vi "VI Tree - appcontrol__ogtk.vi"() -> ()   [LabVIEW 2012]
uses:
  <userlib>/_OpenG.lib/appcontrol/appcontrol.llb/ClassID Names Enum__ogtk.ctl
panel:
  in  "paths":T1
  in  "VI Refnum":refnum<vi>
  in  "Gen Refnum Array 2":refnum<vi>[](array[refnum])
  in  "Gen Refnum Array":refnum<vi>[](array[refnum])
  in  "Gen Refnum":refnum<vi>
  out "ClassID Name":T2=enum."Decoration"
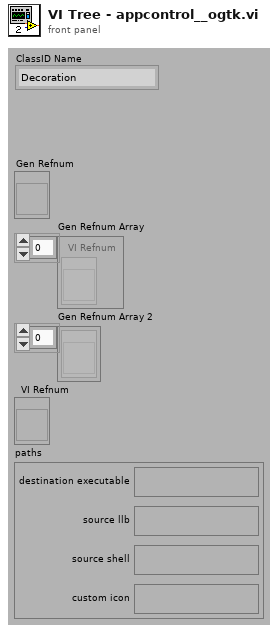
[diagram p1: front panel]
types:
  T1 = cluster{"destination executable":path, "source llb":path, "source shell":path, "custom icon":path}
  T2 = typedef "ClassID Names Enum__ogtk.ctl" = enum32{"0 <undefined>", "1 <undefined>", "2 <undefined>", "Generic", "Decoration", "Text", "Control", "ColorBox", "Boolean", "RefNum", "Variant", "Path", "ListBox", "Table", "Array", "Picture", "ActiveXContainer", "Numeric", "Digital", "NamedNumeric", "ColorRamp", "Slide", "GraphOrChart", "WaveformChart", "WaveformGraph", "IntensityChart", "IntensityGraph", "String", "IOName", "ComboBox", "Cluster", "Panel", "Knob", "NumWithScale", "Ring", "Enum", "GObject", "Plot", "Cursor", "NumericText", "Scale", "ColorScale", "GraphScale", "ColorGraphScale", "TypedRefNum", "OldKnobScale", "MCListbox", "MeasureData", "BVTag", "DAQName", "VISAName", "IVIName", "SlideScale", "TabControl", "Page", "TabArrayTabControl", "ConPane"}
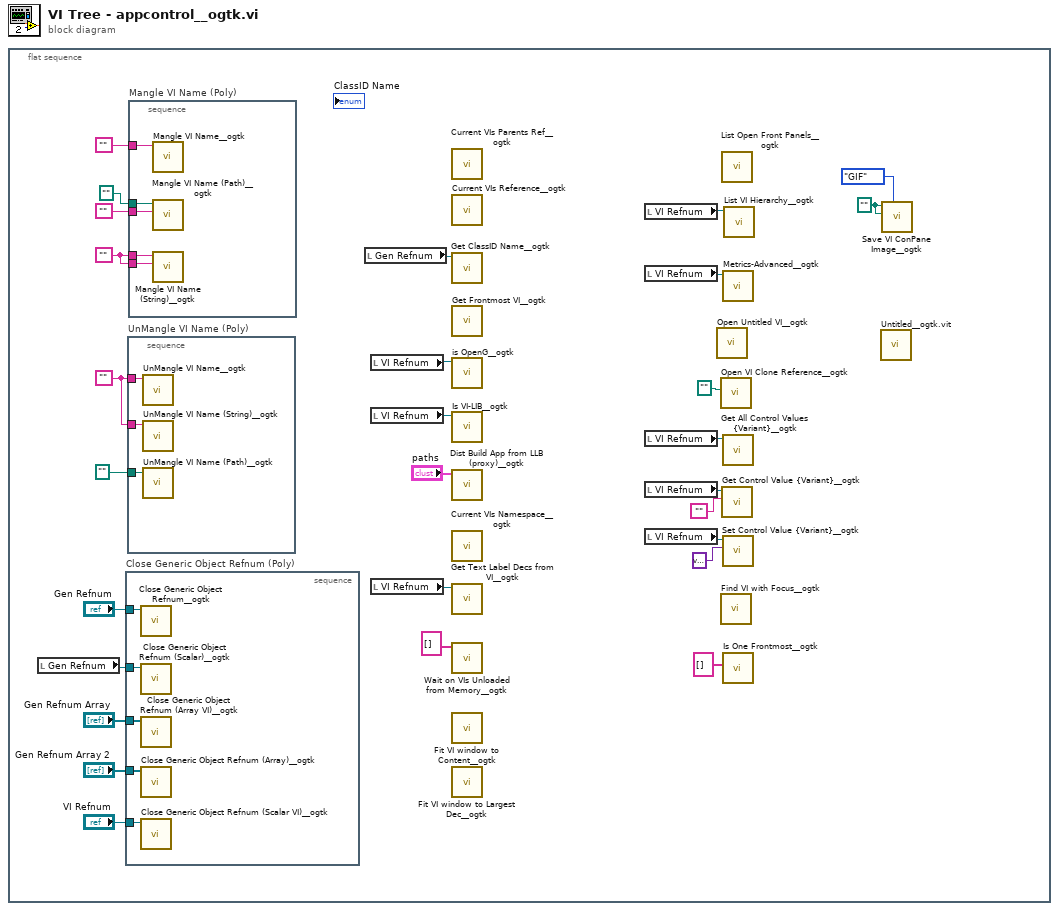
[diagram p0: block diagram]
diagram:
  n1 = flat-sequence {
    frame #0 {
      w2 = path ""
      w18 = ""
      w27 = ""
      n2 = local read "Gen Refnum"() -> (w14:refnum<vi>)
      n3 = stacked-sequence "Close Generic Object Refnum (Poly)" {
        tunnel: "Gen Refnum" -> [w36]
        tunnel: "Gen Refnum Array" -> [w35]
        tunnel: "Gen Refnum Array 2" -> [w34]
        tunnel: "VI Refnum" -> [w33]
        tunnel: w14 -> [w32]
        frame #0 {
          n4 = call-poly <userlib>:"Close Generic Object Refnum__ogtk.vi"("Gen Refnum"=w36) -> ()  [unwired: 10 in, 1 out]
          n5 = call <userlib>:"Close Generic Object Refnum (Scalar)__ogtk.vi"("Gen Refnum"=w32) -> ()  [unwired: 10 in, 1 out]
          n6 = call <userlib>:"Close Generic Object Refnum (Array VI)__ogtk.vi"("Gen Refnum Array"=w35) -> ()  [unwired: 9 in, 2 out]
          n7 = call <userlib>:"Close Generic Object Refnum (Array)__ogtk.vi"("Gen Refnum Array"=w34) -> ()  [unwired: 10 in, 1 out]
          n8 = call <userlib>:"Close Generic Object Refnum (Scalar VI)__ogtk.vi"("VI Refnum"=w33) -> ()  [unwired: 9 in, 2 out]
        }
      }
      n9 = stacked-sequence "UnMangle VI Name (Poly)" {
        tunnel: w27 -> [w31]
        tunnel: path "" -> [w30]
        tunnel: w27 -> [w29]
        frame #0 {
          n10 = call-poly <userlib>:"UnMangle VI Name__ogtk.vi"("Mangled Name"=w29) -> ()  [unwired: 8 in, 3 out]
          n11 = call <userlib>:"UnMangle VI Name (String)__ogtk.vi"("Mangled Name"=w31) -> ()  [unwired: 8 in, 3 out]
          n12 = call <userlib>:"UnMangle VI Name (Path)__ogtk.vi"("Mangled Name"=w30) -> ()  [unwired: 8 in, 3 out]
        }
      }
      n13 = stacked-sequence "Mangle VI Name (Poly)" {
        tunnel: "" -> [w41]
        tunnel: "" -> [w40]
        tunnel: path "" -> [w39]
        tunnel: w18 -> [w38]
        tunnel: w18 -> [w37]
        frame #0 {
          n14 = call-poly <userlib>:"Mangle VI Name__ogtk.vi"("Name"=w41) -> ()  [unwired: 9 in, 2 out]
          n15 = call <userlib>:"Mangle VI Name (Path)__ogtk.vi"("Namespace (\"\": don't mangle)"=w40, "Name"=w39) -> ()  [unwired: 8 in, 2 out]
          n16 = call <userlib>:"Mangle VI Name (String)__ogtk.vi"("Namespace (\"\": don't mangle)"=w37, "Name"=w38) -> ()  [unwired: 8 in, 2 out]
        }
      }
      n17 = local read "Gen Refnum"() -> (w15:refnum<vi>)
      n18 = local read "VI Refnum"() -> (w13:refnum<vi>)
      n19 = local read "VI Refnum"() -> (w12:refnum<vi>)
      n20 = local read "VI Refnum"() -> (w17:refnum<vi>)
      n21 = call <userlib>:"Current VIs Parents Ref__ogtk.vi"() -> ()  [unwired: 2 in, 1 out]
      n22 = call <userlib>:"Current VIs Reference__ogtk.vi"() -> ()  [unwired: 5 in, 1 out]
      n23 = call <userlib>:"Get ClassID Name__ogtk.vi"("Gen Refnum"=w15) -> ()  [unwired: 7 in, 4 out]
      n24 = call <userlib>:"Get Frontmost VI__ogtk.vi"() -> ()  [unwired: 1 out]
      n25 = call <userlib>:"is OpenG__ogtk.vi"("VI reference"=w13) -> ()  [unwired: 8 in, 3 out]
      n26 = call <userlib>:"Is VI-LIB__ogtk.vi"("VI reference"=w12) -> ()  [unwired: 8 in, 3 out]
      n27 = call <userlib>:"Dist Build App from LLB (proxy)__ogtk.vi"("paths"="paths") -> ()  [unwired: 10 in, 1 out]
      n28 = call <userlib>:"Current VIs Namespace__ogtk.vi"() -> ()  [unwired: 5 in, 1 out]
      n29 = call <userlib>:"Get Text Label Decs from VI__ogtk.vi"("VI Refnum"=w17) -> ()  [unwired: 8 in, 3 out]
      n30 = call <userlib>:"Wait on VIs Unloaded from Memory__ogtk.vi"("VIs to Wait on"=string[] [] ("VI names")) -> ()  [unwired: 9 in, 2 out]
      n31 = call <userlib>:"Fit VI window to Content__ogtk.vi"() -> ()  [unwired: 6 in, 2 out]
      n32 = call <userlib>:"Fit VI window to Largest Dec__ogtk.vi"() -> ()  [unwired: 6 in, 2 out]
      n33 = local read "VI Refnum"() -> (w16:refnum<vi>)
      n34 = local read "VI Refnum"() -> (w9:refnum<vi>)
      n35 = local read "VI Refnum"() -> (w7:refnum<vi>)
      n36 = local read "VI Refnum"() -> (w6:refnum<vi>)
      n37 = local read "VI Refnum"() -> (w4:refnum<vi>)
      n38 = call <userlib>:"Open Untitled VI__ogtk.vi"() -> ()  [unwired: 6 in, 2 out]
      n39 = call <userlib>:"Open VI Clone Reference__ogtk.vi"("vi path"=path "") -> ()  [unwired: 9 in, 2 out]
      n40 = call <userlib>:"Find VI with Focus__ogtk.vi"() -> ()  [unwired: 7 in, 5 out]
      n41 = call <userlib>:"List Open Front Panels__ogtk.vi"() -> ()  [unwired: 1 out]
      n42 = call <userlib>:"Get Control Value {Variant}__ogtk.vi"("Control Name"="", "VI Refnum"=w6) -> ()  [unwired: 7 in, 3 out]
      n43 = call <userlib>:"Metrics-Advanced__ogtk.vi"("VI reference"=w9) -> ()  [unwired: 8 in, 3 out]
      n44 = call <userlib>:"Get All Control Values {Variant}__ogtk.vi"("VI Refnum"=w7) -> ()  [unwired: 8 in, 3 out]
      n45 = call <userlib>:"Set Control Value {Variant}__ogtk.vi"("Value"=variant, "VI Refnum"=w4) -> ()  [unwired: 8 in, 2 out]
      n46 = call <userlib>:"Is One Frontmost__ogtk.vi"("VI names"=string[] []) -> ()  [unwired: 7 in, 4 out]
      n47 = call <userlib>:"List VI Hierarchy__ogtk.vi"("VI reference"=w16) -> ()  [unwired: 8 in, 3 out]
      n48 = call <userlib>:"Untitled__ogtk.vit"() -> ()  [unwired: 1 in]
      n49 = call <userlib>:"Save VI ConPane Image__ogtk.vi"("Image Format"=enum32{"PNG", "JPEG", "GIF"}."GIF", "Image File Path"=w2, "VI Path"=w2) -> ()  [unwired: 8 in, 1 out]
    }
  }
